vi "Control_type_change.vi"(11 "IRQ Number":u8) -> ()   [LabVIEW 2017]
uses:
  global.vi
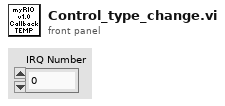
[diagram p1: front panel]
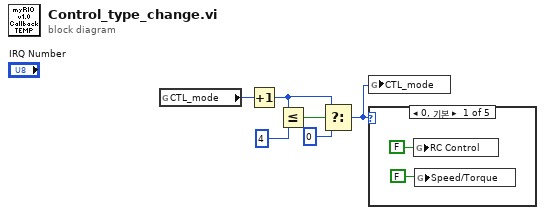
[diagram p0: block diagram]
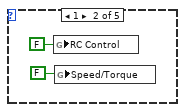
[diagram p2: hidden frame]
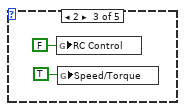
[diagram p3: hidden frame]
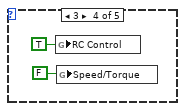
[diagram p4: hidden frame]
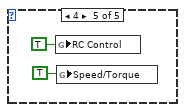
[diagram p5: hidden frame]
diagram:
  n1 = global read "global.vi" "CTL_mode"() -> (w6:u8)
  n2 = Increment(x=w6) -> (x+1=w3:u8)
  n3 = Less Or Equal?(x=w3, y=u8 4) -> (x <= y?=w4:bool)
  n4 = Select(t=w3, s=w4, f=u8 0) -> (s? t:f=w1:u8)
  n5 = global write "global.vi" "CTL_mode"(w1) -> ()
  n6 = case shown="0, 기본" w1 {
    frame 0, Default {
      n7 = global write "global.vi" "RC Control"(FALSE ("RC Control")) -> ()
      n8 = global write "global.vi" "Speed/Torque"(FALSE ("RC Control")) -> ()
    }
    frame 1 {
      n9 = global write "global.vi" "RC Control"(FALSE ("RC Control")) -> ()
      n10 = global write "global.vi" "Speed/Torque"(FALSE ("RC Control")) -> ()
    }
    frame 2 {
      n11 = global write "global.vi" "RC Control"(FALSE ("RC Control")) -> ()
      n12 = global write "global.vi" "Speed/Torque"(TRUE ("RC Control")) -> ()
    }
    frame 3 {
      n13 = global write "global.vi" "RC Control"(TRUE ("RC Control")) -> ()
      n14 = global write "global.vi" "Speed/Torque"(FALSE ("RC Control")) -> ()
    }
    frame 4 {
      n15 = global write "global.vi" "RC Control"(TRUE ("RC Control")) -> ()
      n16 = global write "global.vi" "Speed/Torque"(TRUE ("RC Control")) -> ()
    }
  }
